vi "MTMount_putSample_OSS5.vi"(8 "error in (no error)":errorcluster, 11 "OSS5_Ctl":T1) -> (0 "error out":errorcluster, 2 "function return":i32, 3 "OSS5_Ctl out":T1)   [LabVIEW 2018, in "SALLV_MTMount.lvlib"]
doc: "int MTMount_shm_putSample_OSS5LV(MTMount_OSS5LV *OSS5_Ctl );"
uses:
  SALLV_MTMount.lvlib
  DataTypes/OSS5.ctl
  SALLV_MTMount.so
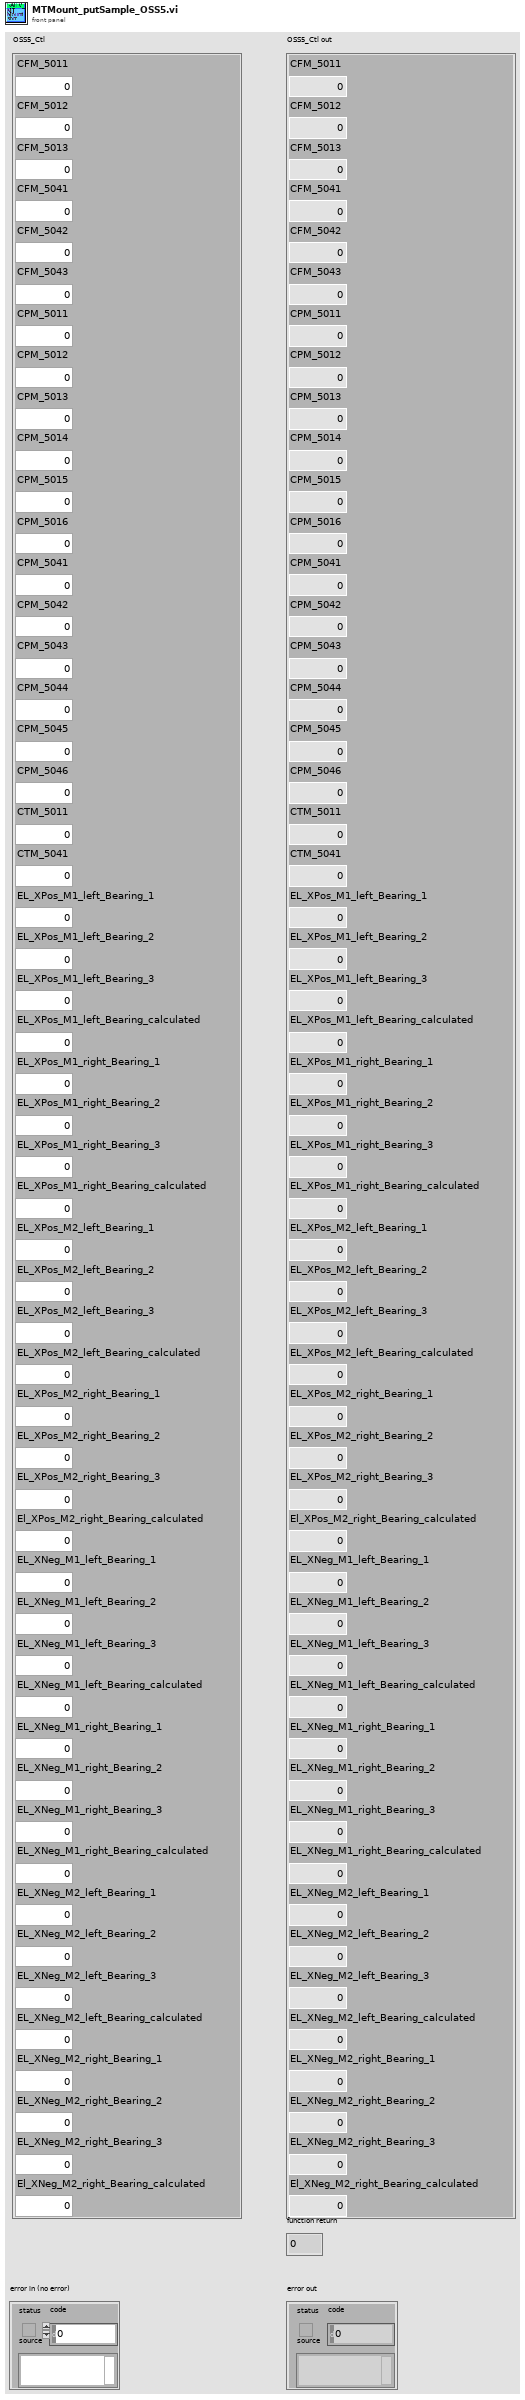
[diagram p1: front panel]
types:
  T1 = typedef "SALLV_MTMount.lvlib/OSS5.ctl" = cluster{"CFM_5011":dbl, "CFM_5012":dbl, "CFM_5013":dbl, "CFM_5041":dbl, "CFM_5042":dbl, "CFM_5043":dbl, "CPM_5011":dbl, "CPM_5012":dbl, "CPM_5013":dbl, "CPM_5014":dbl, "CPM_5015":dbl, "CPM_5016":dbl, "CPM_5041":dbl, "CPM_5042":dbl, "CPM_5043":dbl, "CPM_5044":dbl, "CPM_5045":dbl, "CPM_5046":dbl, "CTM_5011":dbl, "CTM_5041":dbl, "EL_XPos_M1_left_Bearing_1":dbl, "EL_XPos_M1_left_Bearing_2":dbl, "EL_XPos_M1_left_Bearing_3":dbl, "EL_XPos_M1_left_Bearing_calculated":dbl, "EL_XPos_M1_right_Bearing_1":dbl, "EL_XPos_M1_right_Bearing_2":dbl, "EL_XPos_M1_right_Bearing_3":dbl, "EL_XPos_M1_right_Bearing_calculated":dbl, "EL_XPos_M2_left_Bearing_1":dbl, "EL_XPos_M2_left_Bearing_2":dbl, "EL_XPos_M2_left_Bearing_3":dbl, "EL_XPos_M2_left_Bearing_calculated":dbl, "EL_XPos_M2_right_Bearing_1":dbl, "EL_XPos_M2_right_Bearing_2":dbl, "EL_XPos_M2_right_Bearing_3":dbl, "El_XPos_M2_right_Bearing_calculated":dbl, "EL_XNeg_M1_left_Bearing_1":dbl, "EL_XNeg_M1_left_Bearing_2":dbl, "EL_XNeg_M1_left_Bearing_3":dbl, "EL_XNeg_M1_left_Bearing_calculated":dbl, "EL_XNeg_M1_right_Bearing_1":dbl, "EL_XNeg_M1_right_Bearing_2":dbl, "EL_XNeg_M1_right_Bearing_3":dbl, "EL_XNeg_M1_right_Bearing_calculated":dbl, "EL_XNeg_M2_left_Bearing_1":dbl, "EL_XNeg_M2_left_Bearing_2":dbl, "EL_XNeg_M2_left_Bearing_3":dbl, "EL_XNeg_M2_left_Bearing_calculated":dbl, "EL_XNeg_M2_right_Bearing_1":dbl, "EL_XNeg_M2_right_Bearing_2":dbl, "EL_XNeg_M2_right_Bearing_3":dbl, "El_XNeg_M2_right_Bearing_calculated":dbl}
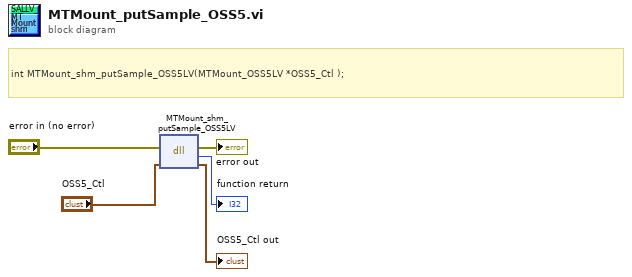
[diagram p0: block diagram]
diagram:
  # "int MTMount_shm_putSample_OSS5LV(MTMount_OSS5LV *OSS5_Ctl );"
  n1 = dll-call lib="home/ttsai/Document/salApiMTMount/SALLV_MTMount/SALLV_MTMount.*" fn="MTMount_shm_putSample_OSS5LV"(error in="error in (no error)", "OSS5_Ctl"="OSS5_Ctl") -> (error out=→"error out":errorcluster, →"function return":i32, "OSS5_Ctl"=→"OSS5_Ctl out":T1)  [unwired: 2 in, 1 out]
